vi "allDictPage.vi"() -> ()   [LabVIEW 2019]
doc: "Use this template to build a producer/consumer design pattern with events to produce queue items. Use this design pattern instead of the User Interface Event Handler pattern for user interfaces when you want to execute code asynchronously in response to an event without slowing the user interface responsiveness."
uses:
  TypeDefs/dictCluster.ctl
  TypeDefs/recDataClust.ctl
  TypeDefs/serialSettings_Global.vi
  <vilib>/Instr/_visa.llb/VISA Configure Serial Port (Instr).vi
  TypeDefs/TCPSettings_Global.vi
  <vilib>/ErrorRing/Error Ring.xnode
panel:
  out "Recieved Data":T1
  out "Consumer Error Out":errorcluster
  out "RecCmdLED":bool caption="Receiving"
  out "TCP Written len":u32
  in  "Send Command TCPIP":bool
  out "UART written count":u32
  out "SendCmdLED":bool caption="Sending"
  out "H2F Frame":string
  in  "Sensor Array":bool[](array[boolean])
  in  "On/Off Data":bool
  out "Read Data":string
  in  "Write Data (Hex)":string
  out "Dictionary":T2
  in  "Select Macro Function":T3(radio)
  in  "Choose Command Type":T4(radio)
  in  "Additional Commands":string(combo)="40"
  in  "Channel Command":string(combo)="30"
  in  "Config & Control Command":string(combo)="20"
  in  "Information Command":string(combo)="10"
  in  "Send Command UART":bool
  in  "stop":bool
  # "DEBUGGING STUFF (Hide! Dont delete)"
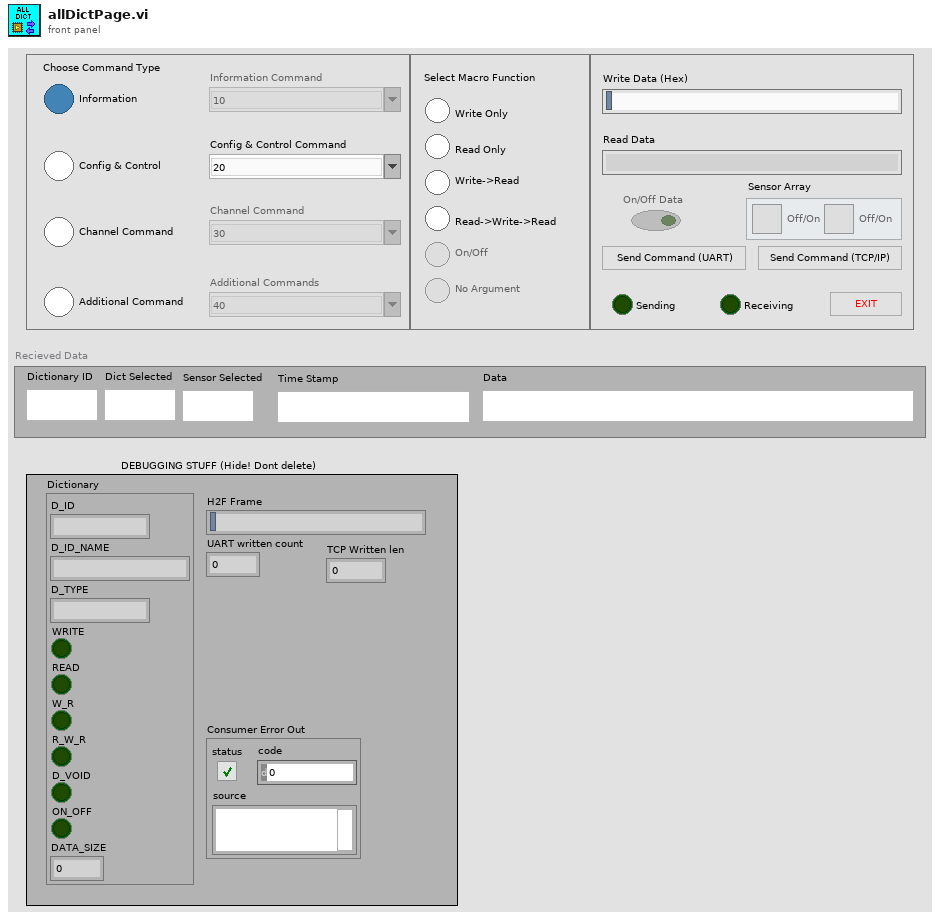
[diagram p1: front panel]
types:
  T1 = typedef "recDataClust.ctl" = cluster{"Dictionary ID":string, "Dict Selected":string, "Sensor Selected":string, "Time Stamp":string, "Data":string}
  T2 = typedef "dictCluster.ctl" = cluster{"D_ID":string, "D_ID_NAME":string, "D_TYPE":string, "WRITE":bool, "READ":bool, "W_R":bool, "R_W_R":bool, "D_VOID":bool, "ON_OFF":bool, "DATA_SIZE":u8}
  T3 = enum32{"No Selection", "WRITE", "READ", "WRITE -> READ", "READ -> WRITE -> READ", "ON/OFF", "NO ARGS"}
  T4 = enum32{"Information", "Config&Control", "Channel", "Additional"}
  T5 = cluster{"VISA resource name":refnum<visa-resource-name>, "baud rate":u32, "data bits":u16, "parity":enum16{"None", "Odd", "Even", "Mark", "Space"}, "stop bits":u16, "flow control":u16}
  T6 = enum8{"Enabled", "Disabled", "Disabled and Grayed Out"}
  T7 = cluster{"D_ID":string, "D_ID_NAME":string, "D_TYPE":string, "WRITE":bool, "READ":bool, "W_R":bool, "R_W_R":bool, "D_VOID":bool, "ON_OFF":bool, "DATA_SIZE":u8}
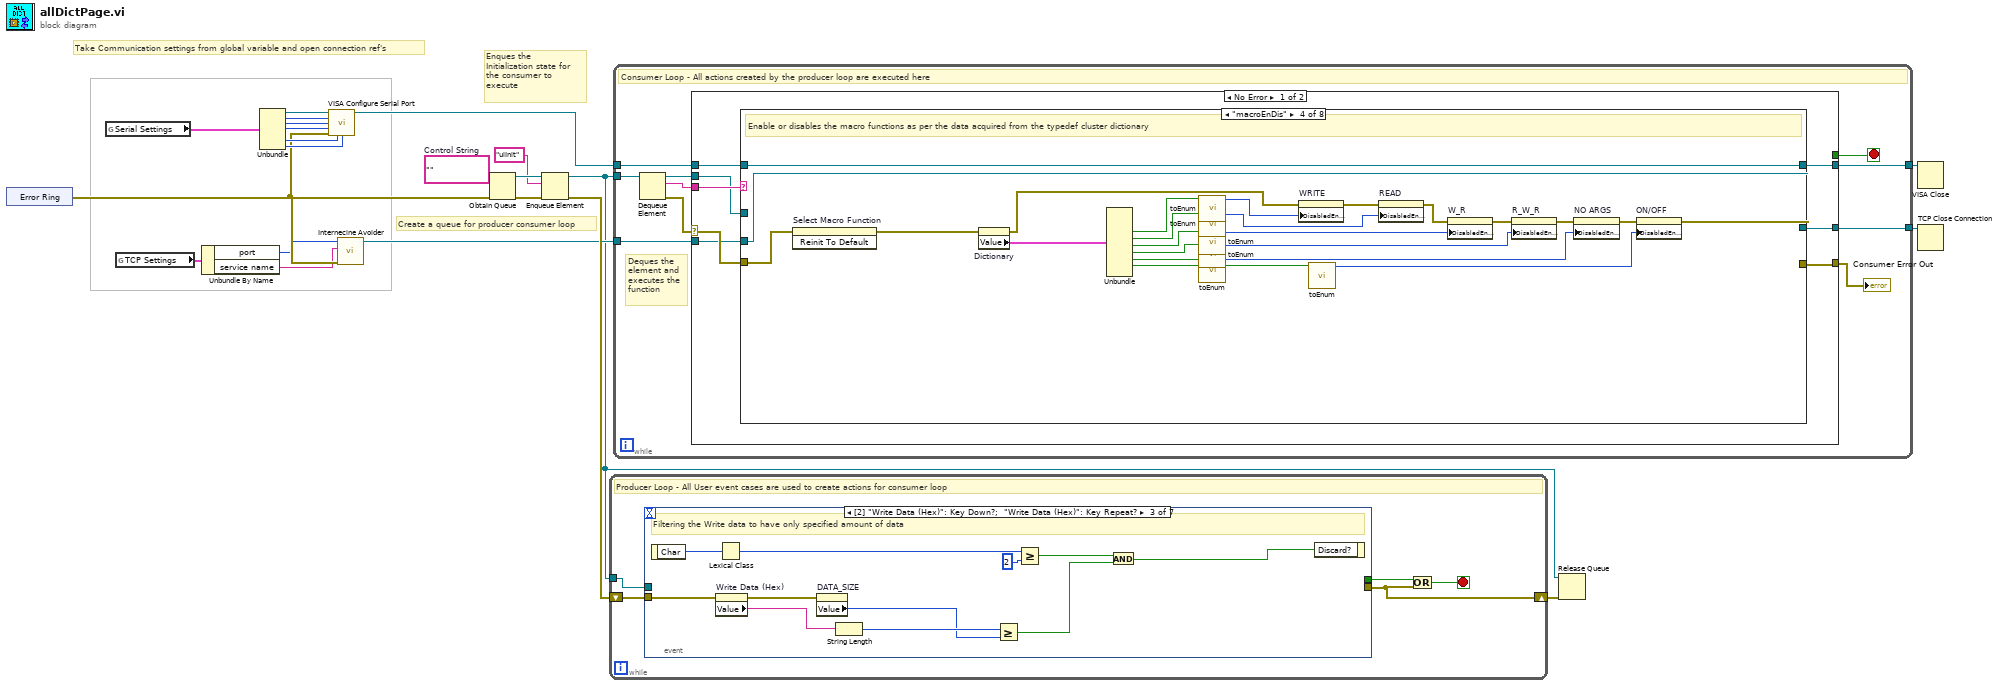
[diagram p0: block diagram]
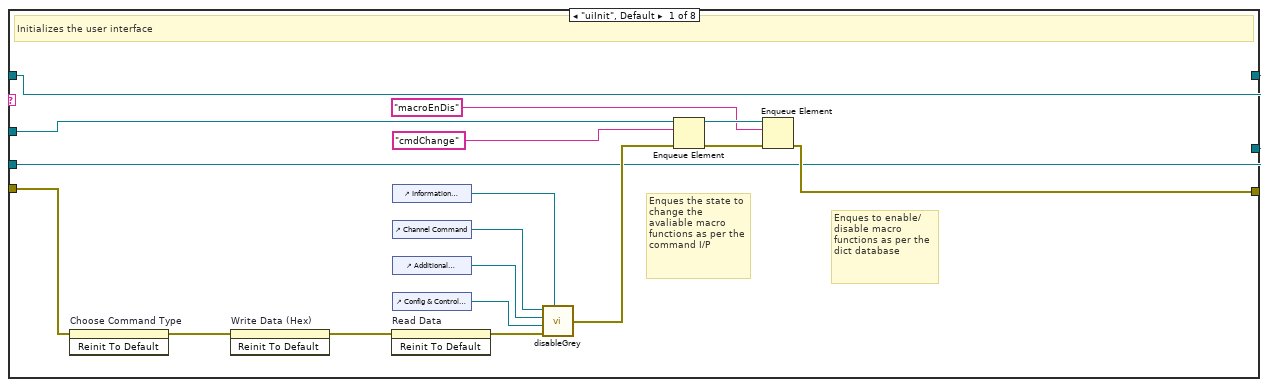
[diagram p2: hidden frame]
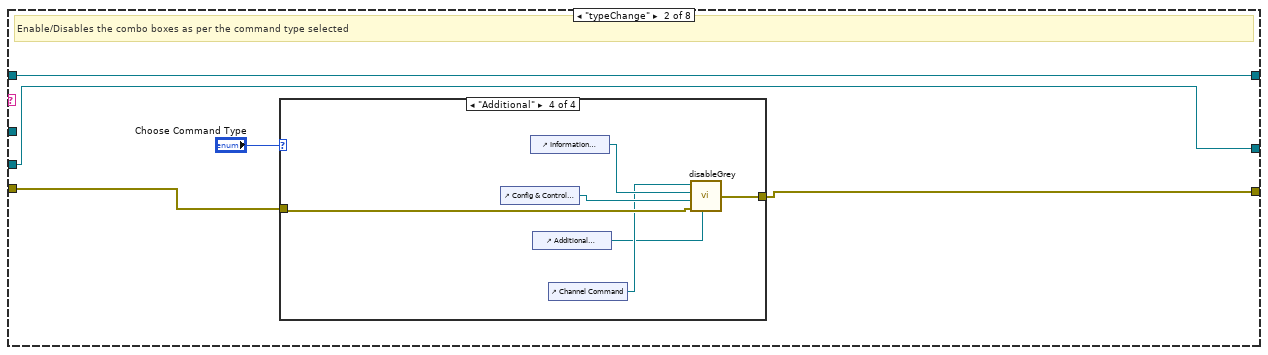
[diagram p3: hidden frame]
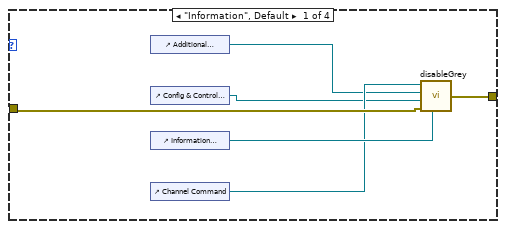
[diagram p4: hidden frame]
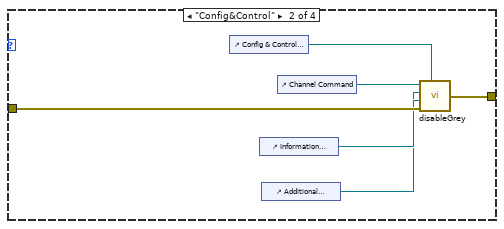
[diagram p5: hidden frame]
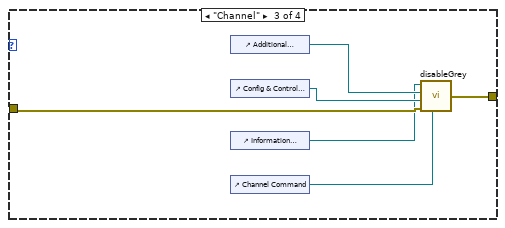
[diagram p6: hidden frame]
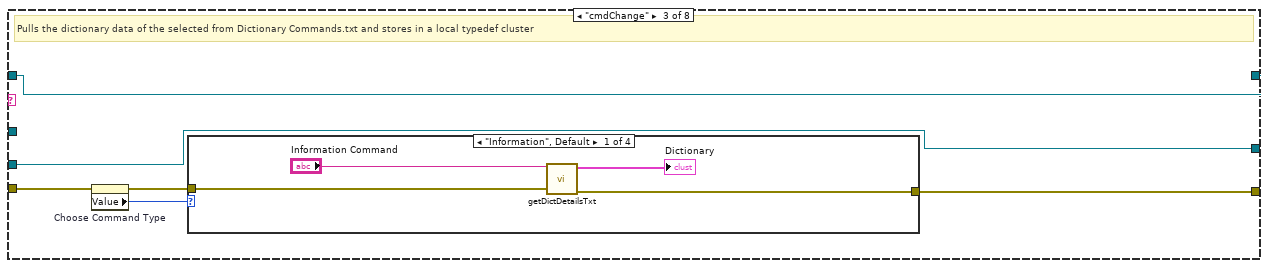
[diagram p7: hidden frame]
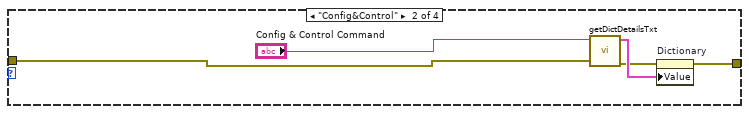
[diagram p8: hidden frame]
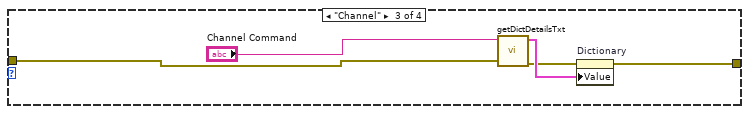
[diagram p9: hidden frame]
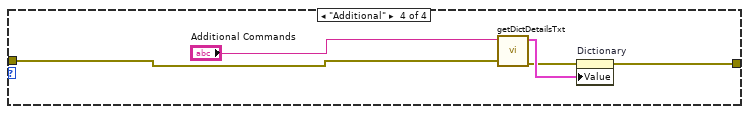
[diagram p10: hidden frame]
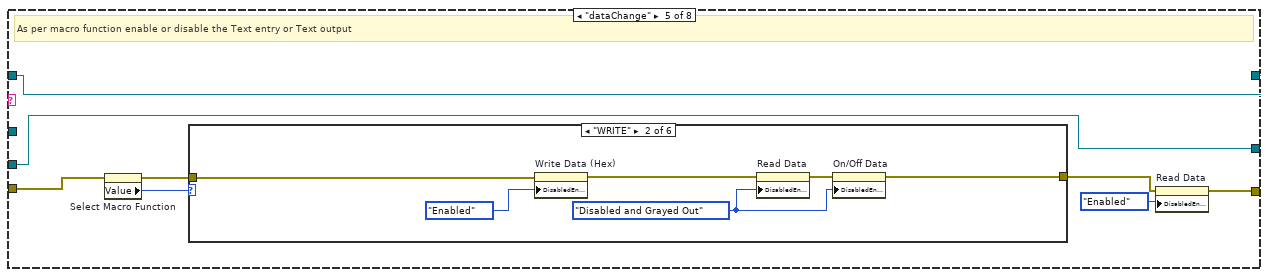
[diagram p11: hidden frame]
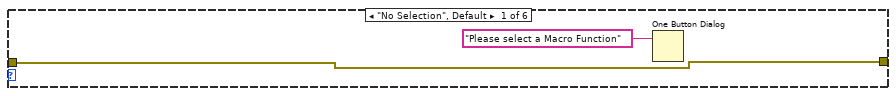
[diagram p12: hidden frame]
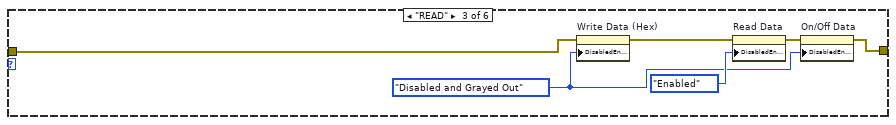
[diagram p13: hidden frame]
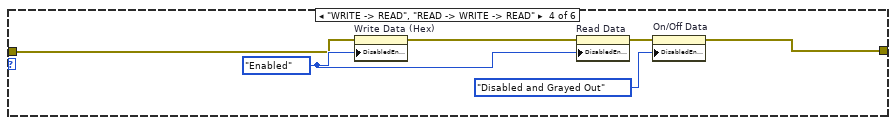
[diagram p14: hidden frame]
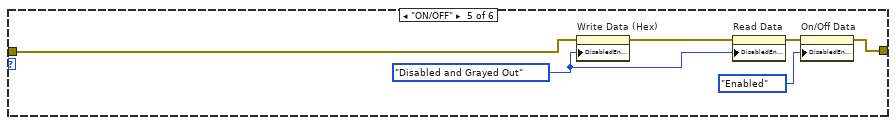
[diagram p15: hidden frame]
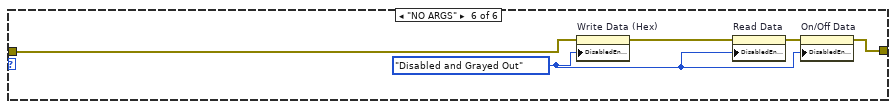
[diagram p16: hidden frame]
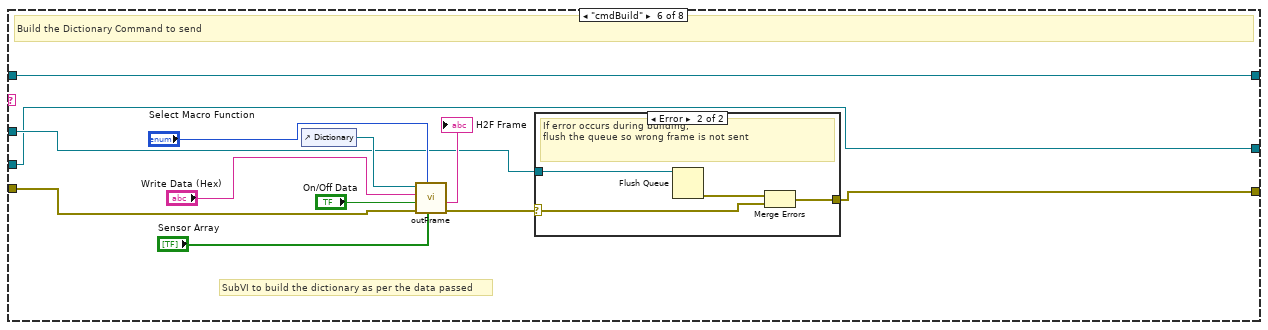
[diagram p17: hidden frame]
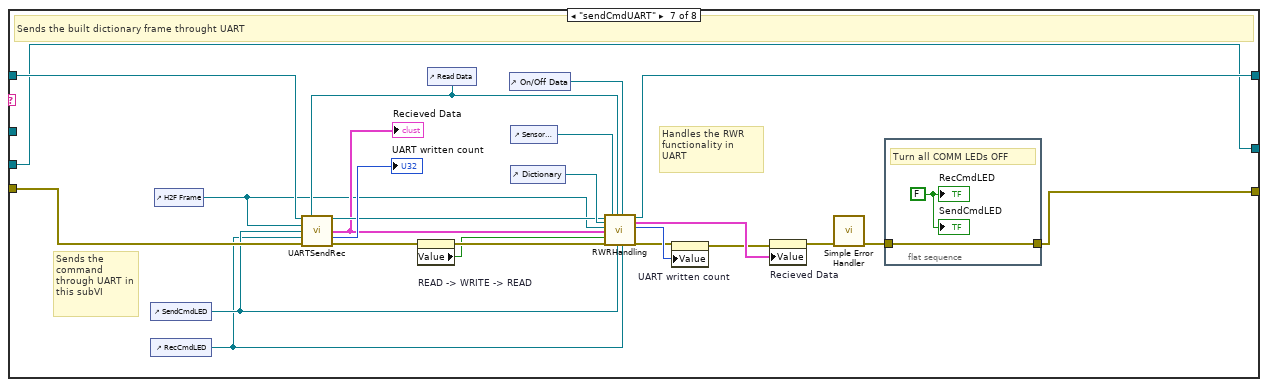
[diagram p19: hidden frame]
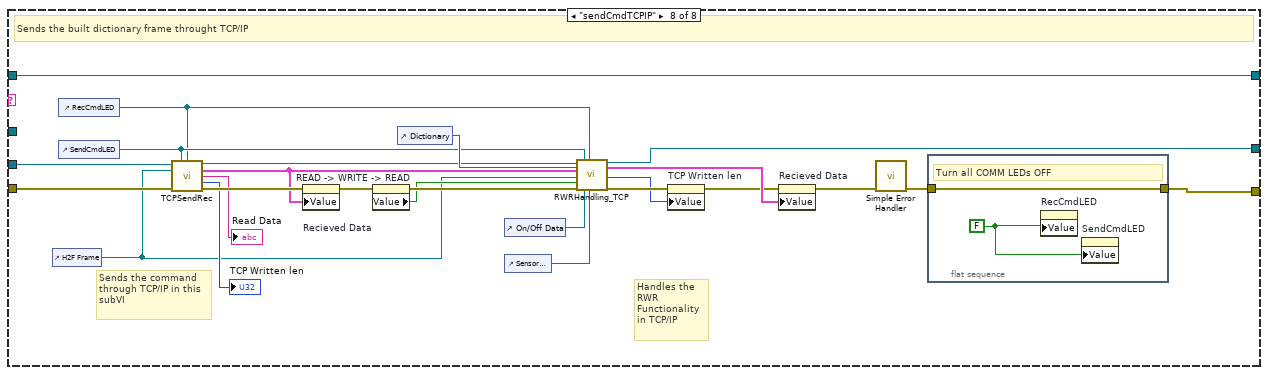
[diagram p20: hidden frame]
diagram:
  w20 = ""  # Control String
  # "Enques the Initialization state for the consumer to execute"
  # "Create a queue for producer consumer loop"
  # "Take Communication settings from global variable and open connection ref's"
  n1 = xnode "Error Ring"() -> ("error out"=w8:errorcluster)
  n2 = global read "serialSettings_Global.vi" "Serial Settings"() -> (w4:T5)
  n3 = global read "TCPSettings_Global.vi" "TCP Settings"() -> (w3:cluster{"service name":string, "port":u16})
  n4 = Unbundle By Name(w3) -> ("port"=w2:u16, "service name"=w1:string)
  n5 = Unbundle(w4) -> ("VISA resource name"=w9:refnum<visa-resource-name>, "baud rate"=w10:u32, "data bits"=w11:u16, "parity"=w12:enum16{"None", "Odd", "Even", "Mark", "Space"}, "stop bits"=w13:u16, "flow control"=w14:u16)
  n6 = call-poly "VISA Configure Serial Port"("VISA resource name"=w9, "baud rate (9600)"=w10, "data bits (8)"=w11, "parity (0:none)"=w12, "error in (no error)"=w8, "stop bits (10: 1 bit)"=w13, "flow control (0:none)"=w14) -> ("VISA resource name out"=w7:refnum<visa-resource-name>)  [unwired: 7 in, 1 out]
  n7 = call <vilib>:"Internecine Avoider.vi"("error in"=w8, "service name"=w1, "port"=w2) -> ("connection ID"=w16:refnum<k5>)  [unwired: 1 in, 7 out]
  n8 = Obtain Queue(element data type=w20, error in (no error)=w8) -> (queue out=w21:refnum<queue>, error out=w19:errorcluster)  [unwired: 3 in, 1 out]
  n9 = Enqueue Element(queue=w21, element="uiInit", error in (no error)=w19) -> (queue out=w15:refnum<queue>, error out=w18:errorcluster)  [unwired: 1 in, 1 out]
  n10 = while {
    shift-right: [w23] -> w22
    shift-left: w18 -> [w26]
    tunnel: w15 -> [w27]
    stop <- w24 stop-if-true
    # "Producer Loop - All User event cases are used to create actions for consumer loop"
    n11 = event shown="[2] \"Write Data (Hex)\": Key Down?;  \"Write Data (Hex)\": Key Repeat?" {
      selector: _ -> [_ _ _ _ _ _ _]
      dyn-events: _ -> [_ _ _ _ _ _ _]
      timeout: _ -> [_ _ _ _ _ _ _]
      tunnel: w27 -> [w34 w41 _ w61 w69 w71 _]
      tunnel: w26 -> [w32 w39 w45 w60 w68 w73 w74]
      tunnel: [w30 w37 _ w55 w66 w72 w74] -> w23
      tunnel: [_ _ _ _ _ _ "stop"] -> w25
      event "Send Command UART": Value Change {
        # "Sends command to build and send command through UART"
        n12 = event-data() -> ()  [unwired: 1 in, 1 out]
        n13 = Enqueue Element(queue=w34, element="cmdBuild", error in (no error)=w32) -> (queue out=w29:refnum<queue>, error out=w33:errorcluster)  [unwired: 1 in, 1 out]
        n14 = Enqueue Element(queue=w29, element="sendCmdUART", error in (no error)=w33) -> (error out=w30:errorcluster)  [unwired: 1 in, 2 out]
      }
      event "Send Command TCPIP": Value Change {
        # "Sends command to build and send command through TCP"
        n15 = event-data() -> ()  [unwired: 1 in, 1 out]
        n16 = Enqueue Element(queue=w41, element="cmdBuild", error in (no error)=w39) -> (queue out=w36:refnum<queue>, error out=w40:errorcluster)  [unwired: 1 in, 1 out]
        n17 = Enqueue Element(queue=w36, element="sendCmdTCPIP", error in (no error)=w40) -> (error out=w37:errorcluster)  [unwired: 1 in, 2 out]
      }
      event "Write Data (Hex)": Key Down?; "Write Data (Hex)": event type 3.0.x8000000b {
        # "Filtering the Write data to have only specified amount of data"
        n18 = event-data() -> ("Char"=w48:i16)  [unwired: 1 in]
        n19 = property on="Write Data (Hex)" class="Str"(error in=w45) -> (error out=w42:errorcluster, "Value"=w44:string)  [unwired: 1 in, 1 out]
        n20 = Lexical Class(1:w48) -> (0:w49:i16)
        n21 = property on="DATA_SIZE" class="DigNum (strict)"(error in=w42) -> ("Value"=w43:u8)  [unwired: 1 in, 2 out]
        n22 = String Length(string=w44) -> (length=w50:i32)
        n23 = Greater Or Equal?(x=w50, y=w43) -> (x >= y?=w51:bool)
        n24 = Greater Or Equal?(x=w49, y=i16 2) -> (x >= y?=w52:bool)
        n25 = And(x=w52, y=w51) -> (x .and. y?=w46:bool)
        n26 = event-data("Discard?"=w46) -> ()  [unwired: 1 in, 1 out]
      }
      event "Choose Command Type": Value Change {
        # "Sends command to consumer loop to enable/disable macro functions as per the User input"
        n27 = event-data() -> ()  [unwired: 1 in, 1 out]
        n28 = Enqueue Element(queue=w61, element="typeChange", error in (no error)=w60) -> (queue out=w57:refnum<queue>, error out=w62:errorcluster)  [unwired: 1 in, 1 out]
        n29 = Enqueue Element(queue=w57, element="cmdChange", error in (no error)=w62) -> (queue out=w54:refnum<queue>, error out=w58:errorcluster)  [unwired: 1 in, 1 out]
        n30 = Enqueue Element(queue=w54, element="macroEnDis", error in (no error)=w58) -> (error out=w55:errorcluster)  [unwired: 1 in, 2 out]
      }
      event "Information Command", "Config & Control Command", "Additional Commands", "Channel Command": Value Change {
        # "Commands selected by the user enable/disable the macro functions"
        n31 = event-data() -> ()  [unwired: 1 in, 1 out]
        n32 = Enqueue Element(queue=w69, element="cmdChange", error in (no error)=w68) -> (queue out=w63:refnum<queue>, error out=w65:errorcluster)  [unwired: 1 in, 1 out]
        n33 = Enqueue Element(queue=w63, element="macroEnDis", error in (no error)=w65) -> (error out=w66:errorcluster)  [unwired: 1 in, 2 out]
      }
      event "Select Macro Function": Value Change {
        # "Sends commands to the C-Loop to enable or disable the Text I/P or O/P"
        n34 = event-data() -> ()  [unwired: 1 in, 1 out]
        n35 = Enqueue Element(queue=w71, element="dataChange", error in (no error)=w73) -> (error out=w72:errorcluster)  [unwired: 1 in, 2 out]
      }
      event "stop": Value Change {
        # "Exits the P-C loop"
        n36 = event-data() -> ()  [unwired: 1 in, 1 out]
      }
    }
    n37 = Or(x=w25, y=w23) -> (x .or. y?=w24:bool)
  }
  n38 = while {
    tunnel: w15 -> [w85]
    tunnel: w16 -> [w80]
    tunnel: w7 -> [w78]
    tunnel: [w77] -> w6
    tunnel: [w76] -> w5
    stop <- w82 stop-if-true
    # "Deques the element and executes the function"
    # "Consumer Loop - All actions created by the producer loop are executed here"
    n39 = Dequeue Element(queue=w85) -> (queue out=w81:refnum<queue>, element=w83:string, error out=w84:errorcluster)  [unwired: 2 in, 1 out]
    n40 = case shown="No Error" w84 {
      selector: w84 -> [w91 w301]
      tunnel: w83 -> [w93 _]
      tunnel: [w92 w301] -> w79
      tunnel: [_ TRUE] -> w82
      tunnel: w81 -> [w90 _]
      tunnel: w80 -> [w89 w298]
      tunnel: w78 -> [w88 w299]
      tunnel: [w87 w299] -> w77
      tunnel: [w86 w298] -> w76
      frame No Error {
        n41 = case shown="\"macroEnDis\"" w93 {
          tunnel: w91 -> [w110 w114 w145 w169 w196 w239 w265 w294]
          tunnel: [w101 w113 w142 w170 w189 w228 w268 w275] -> w92
          tunnel: w90 -> [w103 _ _ _ _ w231 _ _]
          tunnel: w89 -> [w94 w111 w140 w165 w192 w229 w249 w293]
          tunnel: w88 -> [w95 w112 w141 w166 w193 w230 w266 w295]
          tunnel: [w95 w112 w141 w166 w193 w230 w250 w295] -> w87
          tunnel: [w94 w111 w140 w165 w192 w229 w249 w277] -> w86
          frame "uiInit", Default {
            # "Enques to enable/disable macro functions as per the dict database"
            # "Enques the state to change the avaliable macro functions as per the command I/P"
            # "Initializes the user interface"
            n42 = invoke on="Choose Command Type" class="RadioBtnsControl (strict)" method="Reinit To Default"(error in=w110) -> (error out=w98:errorcluster)  [unwired: 2 in, 2 out]
            n43 = invoke on="Write Data (Hex)" class="Str" method="Reinit To Default"(error in=w98) -> (error out=w97:errorcluster)  [unwired: 2 in, 2 out]
            n44 = invoke on="Read Data" class="Str" method="Reinit To Default"(error in=w97) -> (error out=w96:errorcluster)  [unwired: 2 in, 2 out]
            n45 = control-ref of="Information Command"() -> (w109:refnum<vi>)
            n46 = control-ref of="Channel Command"() -> (w108:refnum<vi>)
            n47 = control-ref of="Additional Commands"() -> (w107:refnum<vi>)
            n48 = control-ref of="Config & Control Command"() -> (w106:refnum<vi>)
            n49 = call "disableGrey.vi"("Disable 1"=w108, "Disable 2"=w107, "Disable 3"=w106, "error in (no error)"=w96, "Enable this"=w109) -> ("error out"=w105:errorcluster)
            n50 = Enqueue Element(queue=w103, element="cmdChange", error in (no error)=w105) -> (queue out=w100:refnum<queue>, error out=w104:errorcluster)  [unwired: 1 in, 1 out]
            n51 = Enqueue Element(queue=w100, element="macroEnDis", error in (no error)=w104) -> (error out=w101:errorcluster)  [unwired: 1 in, 2 out]
          }
          frame "typeChange" {
            # "Enable/Disables the combo boxes as per the command type selected"
            n52 = case shown="\"Additional\"" "Choose Command Type" {
              tunnel: w114 -> [w121 w127 w133 w138]
              tunnel: [w116 w126 w132 w139] -> w113
              frame "Information", Default {
                n53 = control-ref of="Additional Commands"() -> (w118:refnum<vi>)
                n54 = control-ref of="Config & Control Command"() -> (w117:refnum<vi>)
                n55 = control-ref of="Information Command"() -> (w120:refnum<vi>)
                n56 = control-ref of="Channel Command"() -> (w119:refnum<vi>)
                n57 = call "disableGrey.vi"("Disable 1"=w119, "Disable 2"=w118, "Disable 3"=w117, "error in (no error)"=w121, "Enable this"=w120) -> ("error out"=w116:errorcluster)
              }
              frame "Config&Control" {
                n58 = control-ref of="Config & Control Command"() -> (w122:refnum<vi>)
                n59 = control-ref of="Information Command"() -> (w125:refnum<vi>)
                n60 = control-ref of="Additional Commands"() -> (w124:refnum<vi>)
                n61 = control-ref of="Channel Command"() -> (w123:refnum<vi>)
                n62 = call "disableGrey.vi"("Disable 1"=w123, "Disable 2"=w124, "Disable 3"=w125, "error in (no error)"=w127, "Enable this"=w122) -> ("error out"=w126:errorcluster)
              }
              frame "Channel" {
                n63 = control-ref of="Additional Commands"() -> (w130:refnum<vi>)
                n64 = control-ref of="Config & Control Command"() -> (w131:refnum<vi>)
                n65 = control-ref of="Information Command"() -> (w129:refnum<vi>)
                n66 = control-ref of="Channel Command"() -> (w128:refnum<vi>)
                n67 = call "disableGrey.vi"("Disable 1"=w129, "Disable 2"=w130, "Disable 3"=w131, "error in (no error)"=w133, "Enable this"=w128) -> ("error out"=w132:errorcluster)
              }
              frame "Additional" {
                n68 = control-ref of="Config & Control Command"() -> (w137:refnum<vi>)
                n69 = control-ref of="Information Command"() -> (w136:refnum<vi>)
                n70 = control-ref of="Additional Commands"() -> (w134:refnum<vi>)
                n71 = control-ref of="Channel Command"() -> (w135:refnum<vi>)
                n72 = call "disableGrey.vi"("Disable 1"=w135, "Disable 2"=w136, "Disable 3"=w137, "error in (no error)"=w138, "Enable this"=w134) -> ("error out"=w139:errorcluster)
              }
            }
          }
          frame "cmdChange" {
            # "Pulls the dictionary data of the selected from Dictionary Commands.txt and stores in a local typedef cluster"
            n73 = property on="Choose Command Type" class="RadioBtnsControl (strict)"(error in=w145) -> (error out=w143:errorcluster, "Value"=w144:T4)  [unwired: 1 in, 1 out]
            n74 = case shown="\"Information\", Default" w144 {
              tunnel: w143 -> [w148 w152 w159 w164]
              tunnel: [w146 w154 w155 w160] -> w142
              frame "Information", Default {
                n75 = call "getDictDetailsTxt.vi"("error constant"=w148, "Dictionary ID Input"="Information Command") -> ("error IO"=w146:errorcluster, "Dictionary"=→"Dictionary":T7)  [unwired: 8 in]
              }
              frame "Config&Control" {
                n76 = call "getDictDetailsTxt.vi"("error constant"=w152, "Dictionary ID Input"="Config & Control Command") -> ("error IO"=w150:errorcluster, "Dictionary"=w151:T7)  [unwired: 8 in]
                n77 = property on="Dictionary" class="Clust (strict)"(error in=w150, "Value"=w151) -> (error out=w154:errorcluster)  [unwired: 1 in, 1 out]
              }
              frame "Channel" {
                n78 = call "getDictDetailsTxt.vi"("error constant"=w159, "Dictionary ID Input"="Channel Command") -> ("error IO"=w156:errorcluster, "Dictionary"=w157:T7)  [unwired: 8 in]
                n79 = property on="Dictionary" class="Clust (strict)"(error in=w156, "Value"=w157) -> (error out=w155:errorcluster)  [unwired: 1 in, 1 out]
              }
              frame "Additional" {
                n80 = call "getDictDetailsTxt.vi"("error constant"=w164, "Dictionary ID Input"="Additional Commands") -> ("error IO"=w161:errorcluster, "Dictionary"=w162:T7)  [unwired: 8 in]
                n81 = property on="Dictionary" class="Clust (strict)"(error in=w161, "Value"=w162) -> (error out=w160:errorcluster)  [unwired: 1 in, 1 out]
              }
            }
          }
          frame "macroEnDis" {
            # "Enable or disables the macro functions as per the data acquired from the typedef cluster dictionary"
            n82 = invoke on="Select Macro Function" class="RadioBtnsControl (strict)" method="Reinit To Default"(error in=w169) -> (error out=w168:errorcluster)  [unwired: 2 in, 2 out]
            n83 = property on="Dictionary" class="Clust (strict)"(error in=w168) -> (error out=w176:errorcluster, "Value"=w188:T2)  [unwired: 1 in, 1 out]
            n84 = Unbundle(w188) -> ("WRITE"=w187:bool, "READ"=w186:bool, "W_R"=w185:bool, "R_W_R"=w184:bool, "D_VOID"=w183:bool, "ON_OFF"=w182:bool)  [unwired: 4 out]
            n85 = call "toEnum.vi"("Instruction"=w187) -> ("Enable/Disable?"=w167:u8)  [unwired: 10 in]
            n86 = call "toEnum.vi"("Instruction"=w186) -> ("Enable/Disable?"=w177:u8)  [unwired: 10 in]
            n87 = call "toEnum.vi"("Instruction"=w185) -> ("Enable/Disable?"=w178:u8)  [unwired: 10 in]
            n88 = call "toEnum.vi"("Instruction"=w184) -> ("Enable/Disable?"=w179:u8)  [unwired: 10 in]
            n89 = call "toEnum.vi"("Instruction"=w183) -> ("Enable/Disable?"=w180:u8)  [unwired: 10 in]
            n90 = property on="WRITE" class="Bool (strict)"(error in=w176, "DisabledEnum"=w167) -> (error out=w175:errorcluster)  [unwired: 1 in, 1 out]
            n91 = call "toEnum.vi"("Instruction"=w182) -> ("Enable/Disable?"=w181:u8)  [unwired: 10 in]
            n92 = property on="READ" class="Bool (strict)"(error in=w175, "DisabledEnum"=w177) -> (error out=w174:errorcluster)  [unwired: 1 in, 1 out]
            n93 = property on="W_R" class="Bool (strict)"(error in=w174, "DisabledEnum"=w178) -> (error out=w173:errorcluster)  [unwired: 1 in, 1 out]
            n94 = property on="R_W_R" class="Bool (strict)"(error in=w173, "DisabledEnum"=w179) -> (error out=w172:errorcluster)  [unwired: 1 in, 1 out]
            n95 = property on="NO ARGS" class="Bool (strict)"(error in=w172, "DisabledEnum"=w180) -> (error out=w171:errorcluster)  [unwired: 1 in, 1 out]
            n96 = property on="ON/OFF" class="Bool (strict)"(error in=w171, "DisabledEnum"=w181) -> (error out=w170:errorcluster)  [unwired: 1 in, 1 out]
          }
          frame "dataChange" {
            # "As per macro function enable or disable the Text entry or Text output"
            n97 = property on="Select Macro Function" class="RadioBtnsControl (strict)"(error in=w196) -> (error out=w194:errorcluster, "Value"=w195:T3)  [unwired: 1 in, 1 out]
            n98 = case shown="\"WRITE\"" w195 {
              tunnel: w194 -> [w197 w202 w206 w212 w218 w224]
              tunnel: [w197 w201 w205 w211 w217 w223] -> w191
              frame "No Selection", Default {
                n99 = One Button Dialog(message="Please select a Macro Function") -> ()  [unwired: 1 in, 1 out]
              }
              frame "WRITE" {
                w199 = T6."Disabled and Grayed Out" ("Disabled")
                n100 = property on="Write Data (Hex)" class="Str"(error in=w202, "DisabledEnum"=T6."Enabled" ("Disabled")) -> (error out=w204:errorcluster)  [unwired: 1 in, 1 out]
                n101 = property on="Read Data" class="Str"(error in=w204, "DisabledEnum"=w199) -> (error out=w203:errorcluster)  [unwired: 1 in, 1 out]
                n102 = property on="On/Off Data" class="Bool (strict)"(error in=w203, "DisabledEnum"=w199) -> (error out=w201:errorcluster)  [unwired: 1 in, 1 out]
              }
              frame "READ" {
                w207 = T6."Disabled and Grayed Out" ("Disabled")
                n103 = property on="Write Data (Hex)" class="Str"(error in=w206, "DisabledEnum"=w207) -> (error out=w210:errorcluster)  [unwired: 1 in, 1 out]
                n104 = property on="Read Data" class="Str"(error in=w210, "DisabledEnum"=T6."Enabled" ("Disabled")) -> (error out=w209:errorcluster)  [unwired: 1 in, 1 out]
                n105 = property on="On/Off Data" class="Bool (strict)"(error in=w209, "DisabledEnum"=w207) -> (error out=w205:errorcluster)  [unwired: 1 in, 1 out]
              }
              frame "WRITE -> READ", "READ -> WRITE -> READ" {
                w213 = T6."Enabled" ("Disabled")
                n106 = property on="Write Data (Hex)" class="Str"(error in=w212, "DisabledEnum"=w213) -> (error out=w216:errorcluster)  [unwired: 1 in, 1 out]
                n107 = property on="Read Data" class="Str"(error in=w216, "DisabledEnum"=w213) -> (error out=w215:errorcluster)  [unwired: 1 in, 1 out]
                n108 = property on="On/Off Data" class="Bool (strict)"(error in=w215, "DisabledEnum"=T6."Disabled and Grayed Out" ("Disabled")) -> (error out=w211:errorcluster)  [unwired: 1 in, 1 out]
              }
              frame "ON/OFF" {
                w220 = T6."Disabled and Grayed Out" ("Disabled")
                n109 = property on="Write Data (Hex)" class="Str"(error in=w218, "DisabledEnum"=w220) -> (error out=w222:errorcluster)  [unwired: 1 in, 1 out]
                n110 = property on="Read Data" class="Str"(error in=w222, "DisabledEnum"=w220) -> (error out=w221:errorcluster)  [unwired: 1 in, 1 out]
                n111 = property on="On/Off Data" class="Bool (strict)"(error in=w221, "DisabledEnum"=T6."Enabled" ("Disabled")) -> (error out=w217:errorcluster)  [unwired: 1 in, 1 out]
              }
              frame "NO ARGS" {
                w225 = T6."Disabled and Grayed Out" ("Disabled")
                n112 = property on="Write Data (Hex)" class="Str"(error in=w224, "DisabledEnum"=w225) -> (error out=w227:errorcluster)  [unwired: 1 in, 1 out]
                n113 = property on="Read Data" class="Str"(error in=w227, "DisabledEnum"=w225) -> (error out=w226:errorcluster)  [unwired: 1 in, 1 out]
                n114 = property on="On/Off Data" class="Bool (strict)"(error in=w226, "DisabledEnum"=w225) -> (error out=w223:errorcluster)  [unwired: 1 in, 1 out]
              }
            }
            n115 = property on="Read Data" class="Str"(error in=w191, "DisabledEnum"=T6."Enabled" ("Disabled")) -> (error out=w189:errorcluster)  [unwired: 1 in, 1 out]
          }
          frame "cmdBuild" {
            # "SubVI to build the dictionary as per the data passed"
            # "Build the Dictionary Command to send"
            n116 = control-ref of="Dictionary"() -> (w235:refnum<vi>)
            n117 = call "outFrame.vi"("Sensor Array"="Sensor Array", "Select Macro Function"="Select Macro Function", "error in (no error)"=w239, "On/Off Data"="On/Off Data", "Write Data (HEX)"="Write Data (Hex)", "Cluster in"=w235) -> ("error out"=w232:errorcluster, "H2F Frame"=→"H2F Frame":string)  [unwired: 4 in]
            n118 = case shown="Error" w232 {
              selector: w232 -> [w240 w241]
              tunnel: [w240 w243] -> w228
              tunnel: w231 -> [_ w244]
              frame No Error {
                # "No error, go ahead with the loop"
              }
              frame Error {
                # "If error occurs during building; \nflush the queue so wrong frame is not sent"
                n119 = Flush Queue(queue=w244) -> (error out=w242:errorcluster)  [unwired: 1 in, 2 out]
                n120 = Merge Errors(w242, w241) -> (w243:errorcluster)
              }
            }
          }
          frame "sendCmdUART" {
            # "Handles the RWR functionality in UART"
            # "Sends the command through UART in this subVI"
            # "Sends the built dictionary frame throught UART"
            n121 = control-ref of="SendCmdLED"() -> (w248:refnum<vi>)
            n122 = control-ref of="RecCmdLED"() -> (w247:refnum<vi>)
            n123 = control-ref of="H2F Frame"() -> (w246:refnum<vi>)
            n124 = control-ref of="Read Data"() -> (w251:refnum<vi>)
            n125 = call "UARTSendRec.vi"("VISA resource name in"=w266, "Read Data Ref"=w251, "H2F Frame Ref"=w246, "Send LED Ref"=w248, "Rec LED Ref"=w247, "error in (no error)"=w265) -> ("VISA resource name out"=w259:refnum<visa-resource-name>, "Recieved Data"=w252:T1, "UART written count"=→"UART written count":u32, "error out"=w264:errorcluster)  [unwired: 6 in]
            "Recieved Data" <- w252
            n126 = property on="READ -> WRITE -> READ" class="Bool (strict)"(error in=w264) -> (error out=w262:errorcluster, "Value"=w261:bool)  [unwired: 1 in, 1 out]
            n127 = control-ref of="On/Off Data"() -> (w245:refnum<vi>)
            n128 = control-ref of="Sensor Array"() -> (w253:refnum<vi>)
            n129 = control-ref of="Dictionary"() -> (w260:refnum<vi>)
            n130 = call "RWRHandling.vi"("VISA in"=w259, "Dictionary"=w260, "H2F Frame"=w246, "Recieved Data"=w252, "RWR?"=w261, "error in (no error)"=w262, "SensorArr Ref"=w253, "Read Data"=w251, "SendCmdLED"=w248, "On/Off Data Ref"=w245, "RecCmdLED"=w247) -> ("VISA Refnum out"=w250:refnum<visa-resource-name>, "Recieved Data Out"=w258:T1, "UART written count"=w257:u32, "error out"=w256:errorcluster)  [unwired: 5 in]
            n131 = property on="UART written count" class="DigNum (strict)"(error in=w256, "Value"=w257) -> (error out=w255:errorcluster)  [unwired: 1 in, 1 out]
            n132 = property on="Recieved Data" class="Clust (strict)"(error in=w255, "Value"=w258) -> (error out=w254:errorcluster)  [unwired: 1 in, 1 out]
            n133 = call <vilib>:"Simple Error Handler.vi"("error in (no error)"=w254) -> ("error out"=w267:errorcluster)  [unwired: 4 in, 4 out]
            n134 = flat-sequence {
              tunnel: [w270] -> w268
              tunnel: w267 -> [w270]
              frame #0 {
                w269 = FALSE ("Sending Command")
                # "Turn all COMM LEDs OFF"
                "SendCmdLED" <- w269
                "RecCmdLED" <- w269
              }
            }
          }
          frame "sendCmdTCPIP" {
            # "Handles the RWR Functionality in TCP/IP"
            # "Sends the command through TCP/IP in this subVI"
            # "Sends the built dictionary frame throught TCP/IP"
            n135 = control-ref of="H2F Frame"() -> (w274:refnum<vi>)
            n136 = control-ref of="RecCmdLED"() -> (w271:refnum<vi>)
            n137 = control-ref of="SendCmdLED"() -> (w272:refnum<vi>)
            n138 = call "TCPSendRec.vi"("TCP Conn"=w293, "SendLEDRef"=w272, "RecLEDRef"=w271, "H2F Frame Ref"=w274, "error in (no error)"=w294) -> ("TCP Network Connection out"=w283:refnum<k5>, "Bifurcated Recieved Data"=w284:T1, "Recieved Frame"=→"Read Data":string, "TCP Written Bytes"=→"TCP Written len":i32, "error out"=w292:errorcluster)  [unwired: 6 in]
            n139 = property on="Recieved Data" class="Clust (strict)"(error in=w292, "Value"=w284) -> (error out=w289:errorcluster)  [unwired: 1 in, 1 out]
            n140 = property on="READ -> WRITE -> READ" class="Bool (strict)"(error in=w289) -> (error out=w286:errorcluster, "Value"=w285:bool)  [unwired: 1 in, 1 out]
            n141 = control-ref of="Dictionary"() -> (w288:refnum<vi>)
            n142 = control-ref of="On/Off Data"() -> (w287:refnum<vi>)
            n143 = control-ref of="Sensor Array"() -> (w273:refnum<vi>)
            n144 = call "RWRHandling_TCP.vi"("TCP Conn"=w283, "Dictionary"=w288, "Recieved Data"=w284, "H2F Frame"=w274, "RWR?"=w285, "error in (no error)"=w286, "SendCmdLED"=w272, "On/Off Data Ref"=w287, "RecCmdLED"=w271, "SensorArr Ref"=w273) -> ("TCP Network Connection out"=w277:refnum<k5>, "Bifurcated Recieved Data Out"=w282:T1, "TCP written count"=w279:u32, "error out"=w281:errorcluster)  [unwired: 5 in, 1 out]
            n145 = property on="TCP Written len" class="DigNum (strict)"(error in=w281, "Value"=w279) -> (error out=w280:errorcluster)  [unwired: 1 in, 1 out]
            n146 = property on="Recieved Data" class="Clust (strict)"(error in=w280, "Value"=w282) -> (error out=w278:errorcluster)  [unwired: 1 in, 1 out]
            n147 = call <vilib>:"Simple Error Handler.vi"("error in (no error)"=w278) -> ("error out"=w276:errorcluster)  [unwired: 4 in, 4 out]
            n148 = flat-sequence {
              tunnel: w276 -> [w296]
              tunnel: [w296] -> w275
              frame #0 {
                w297 = FALSE
                # "Turn all COMM LEDs OFF"
                n149 = property on="RecCmdLED" class="Bool (strict)"("Value"=w297) -> ()  [unwired: 2 in, 2 out]
                n150 = property on="SendCmdLED" class="Bool (strict)"("Value"=w297) -> ()  [unwired: 2 in, 2 out]
              }
            }
          }
        }
      }
      frame Error {
        # "Return true in any case that should stop the loop."
        # "Error Occured so stop the loop"
      }
    }
    "Consumer Error Out" <- w79
  }
  n151 = Release Queue(queue=w15, error in (no error)=w22) -> ()  [unwired: 1 in, 3 out]
  n152 = VISA Close(VISA resource name=w6) -> ()  [unwired: 1 in, 1 out]
  n153 = TCP Close Connection(connection ID=w5) -> ()  [unwired: 1 in, 3 out]
